vi "V7310.Position.Set.vi"(6 "timeout ms (5000)":i32=5000, 8 "error in":errorcluster, 10 "Position":cluster{"X":dbl, "Y":dbl}, 11 "Connection in":refnum<k5>) -> (0 "error out":errorcluster, 3 "Connection out":refnum<k5>)   [LabVIEW 2016]
uses:
  LowLevel/V7310.Commands.ctl
panel:
  out "Data out":string
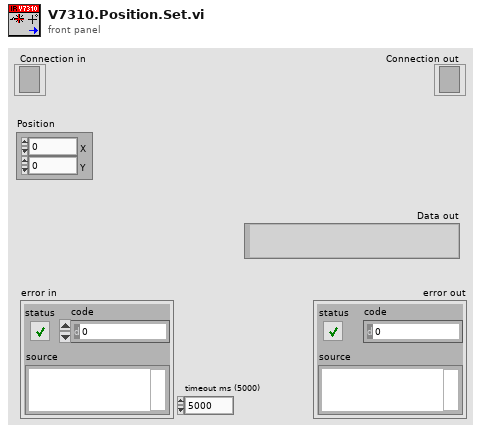
[diagram p1: front panel]
types:
  T1 = typedef "V7310.Commands.ctl" = enum16{"Start", "Stop", "GetStatus", "GetVarNames", "GetJobNames", "SetJob", "GetJob", "SetVars", "GetVars", "SetLayoutPosition", "SetRotation", "GetMessageID", "GetMessages", "ConfirmMessages", "DeleteMessages", "SetRTC", "GetRTC", "SetVarPosition", "SetIntensity", "GetIntensity", "SetStartTriggerDelay", "GetStartTriggerDelay", "SetStopTriggerDelay", "GetStopTriggerDelay", "SetConsecutiveTriggerDelay", "GetConsecutiveTriggerDelay", "SetMarkSpeed", "GetMarkSpeed"}
  T2 = typedef "V7310.ErrorLevels.ctl" = enum16{"OK", "Warning", "Error"}
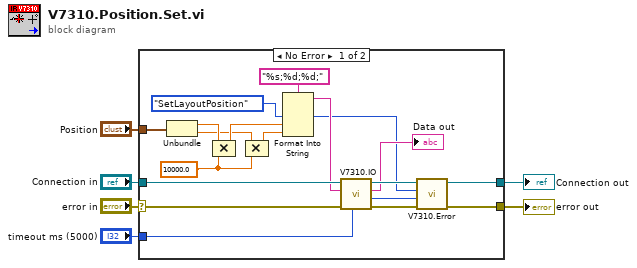
[diagram p0: block diagram]
diagram:
  n1 = case shown="No Error" "error in" {
    selector: "error in" -> [w21 w24]
    tunnel: "Connection in" -> [w22 w25]
    tunnel: [w23 w25] -> w5
    tunnel: "timeout ms (5000)" -> [w20 _]
    tunnel: [w15 w24] -> w2
    tunnel: "Position" -> [w14 _]
    frame No Error {
      w10 = 10000.0 ("y")
      w7 = V7310.Commands."SetLayoutPosition" ("Cmd")
      n2 = Unbundle(w14) -> ("X"=w12:dbl, "Y"=w9:dbl)
      n3 = Compound Arithmetic op=MULTIPLY(w12, w10) -> (w11:dbl)
      n4 = Compound Arithmetic op=MULTIPLY(w9, w10) -> (w8:dbl)
      n5 = Format Into String(format string="%s;%d;%d;", w7, w11, w8) -> (resulting string=w18:string)  [unwired: 2 in, 1 out]
      n6 = call "V7310.IO.vi"("timeout ms (5000)"=w20, "error in"=w21, "Data in"=w18, "Connection in"=w22) -> ("error out"=w16:errorcluster, "Error Level"=w17:T2, "Data out"=→"Data out":string, "Connection out"=w23:refnum<k5>)  [unwired: 4 in]
      n7 = call "V7310.Error.vi"("error in"=w16, "Error Level"=w17, "Cmd"=w7) -> ("error out"=w15:errorcluster)  [unwired: 8 in]
    }
    frame Error {
    }
  }
  "Connection out" <- w5
  "error out" <- w2
